vi "Config Measure Average.vi"(0 "VISA resource name":refnum<visa-resource-name>, 5 "Average (F: OFF)":bool, 7 "Average Count (0: 2)":u16(ring) items=["2", "4", "8", "16", "32", "64"], 11 "error in (no error)":errorcluster) -> (4 "VISA resource name out":refnum<visa-resource-name>, 15 "error out":errorcluster)   [LabVIEW 2013, in "Yokogawa.lvlib" / "Yokogawa PZ4000.lvlib"]
doc: "This VI sends the Average group command to the PZ4000 series."
uses:
  Yokogawa PZ4000.lvlib
panel:
  # "ON\nOFF"
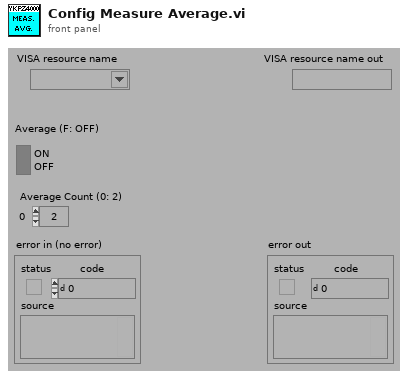
[diagram p1: front panel]
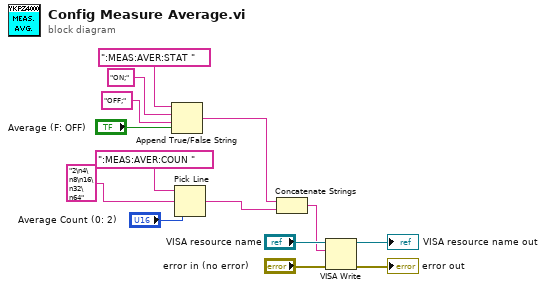
[diagram p0: block diagram]
diagram:
  n1 = Append True/False String(1:"Average (F: OFF)", 2:"OFF;", 3:"ON;", 4:":MEAS:AVER:STAT ") -> (0:w3:string)
  n2 = Pick Line(string ("")=":MEAS:AVER:COUN ", multi-line string="2\n4\n8\n16\n32\n64", line index="Average Count (0: 2)") -> (output string=w2:string)
  n3 = Concatenate Strings(w3, w2) -> (w1:string)
  n4 = VISA Write(VISA resource name="VISA resource name", write buffer=w1, error in (no error)="error in (no error)") -> (VISA resource name out=→"VISA resource name out":refnum<visa-resource-name>, error out=→"error out":errorcluster)  [unwired: 1 out]
